vi "set_electrodes_init (SubVI).vi"(0 "Tot Electrode Arr":dbl[](array[numeric]), 5 "electrodes task 2":refnum<k21>, 9 "electrodes error":errorcluster, 11 "electrodes reference":refnum<vi>) -> (4 "electrode arr":dbl[][](array[numeric]), 6 "electrodes task":refnum<k21>, 15 "electrodes task error":errorcluster)   [LabVIEW 2018]
uses:
  <resource>/objmgr/daqmx.rc
  <vilib>/measure/NI_MABase.lvlib
panel:
  out "SampClk.Rate":dbl
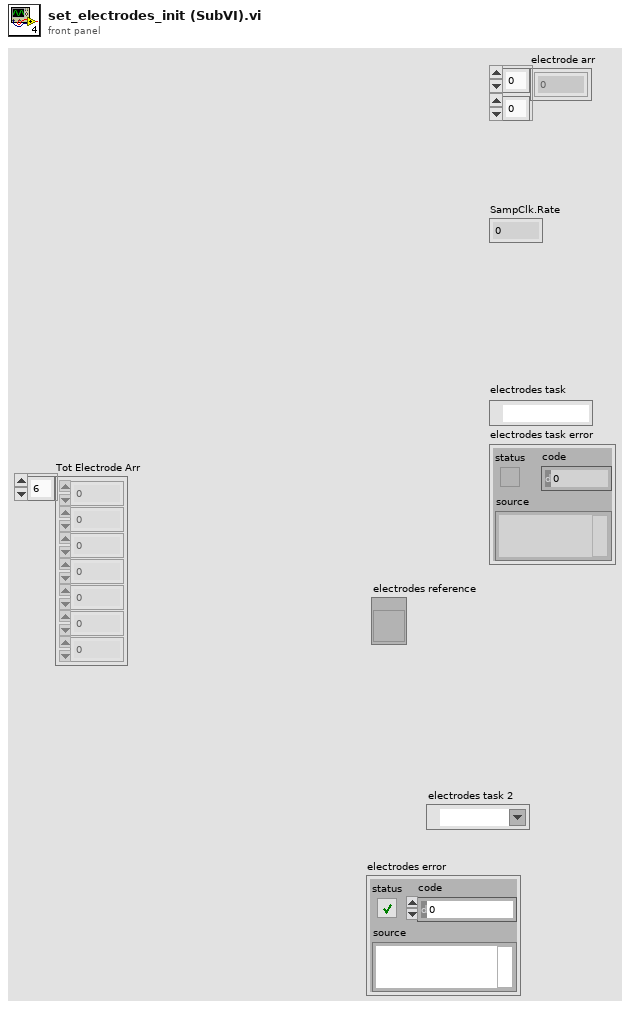
[diagram p1: front panel]
types:
  T1 = cluster{"DC volts (V):\n":dbl[], "Electrode to sweep:":i32, "start volt (V)":ext, "stop volt (V) ":ext, "# V Steps":i32, "start freq (Hz)":ext, "stop freq (Hz) ":ext, "# F steps":i32, "start DC (V)":ext, "stop DC (V)":ext, "# DC steps ":i32, "Digitize electrode\ndrives?":bool, "Sweep electrode?":bool, "Add 0.5*V DC \noffset for amp?":bool, "Use electrode \nconfig file?":bool, "Path":path, "Use arbitrary\nforce func?":bool, "Voltage vs pos file":path, "Use Arbitrary elec drive":bool, "Elec Drive File":path, "Filter Elecs?":bool, "Filter Cantilever?":bool, "Control DDS":bool}
  T2 = enum16{"Sine Wave", "Triangle Wave", "Square Wave", "Sawtooth Wave"}
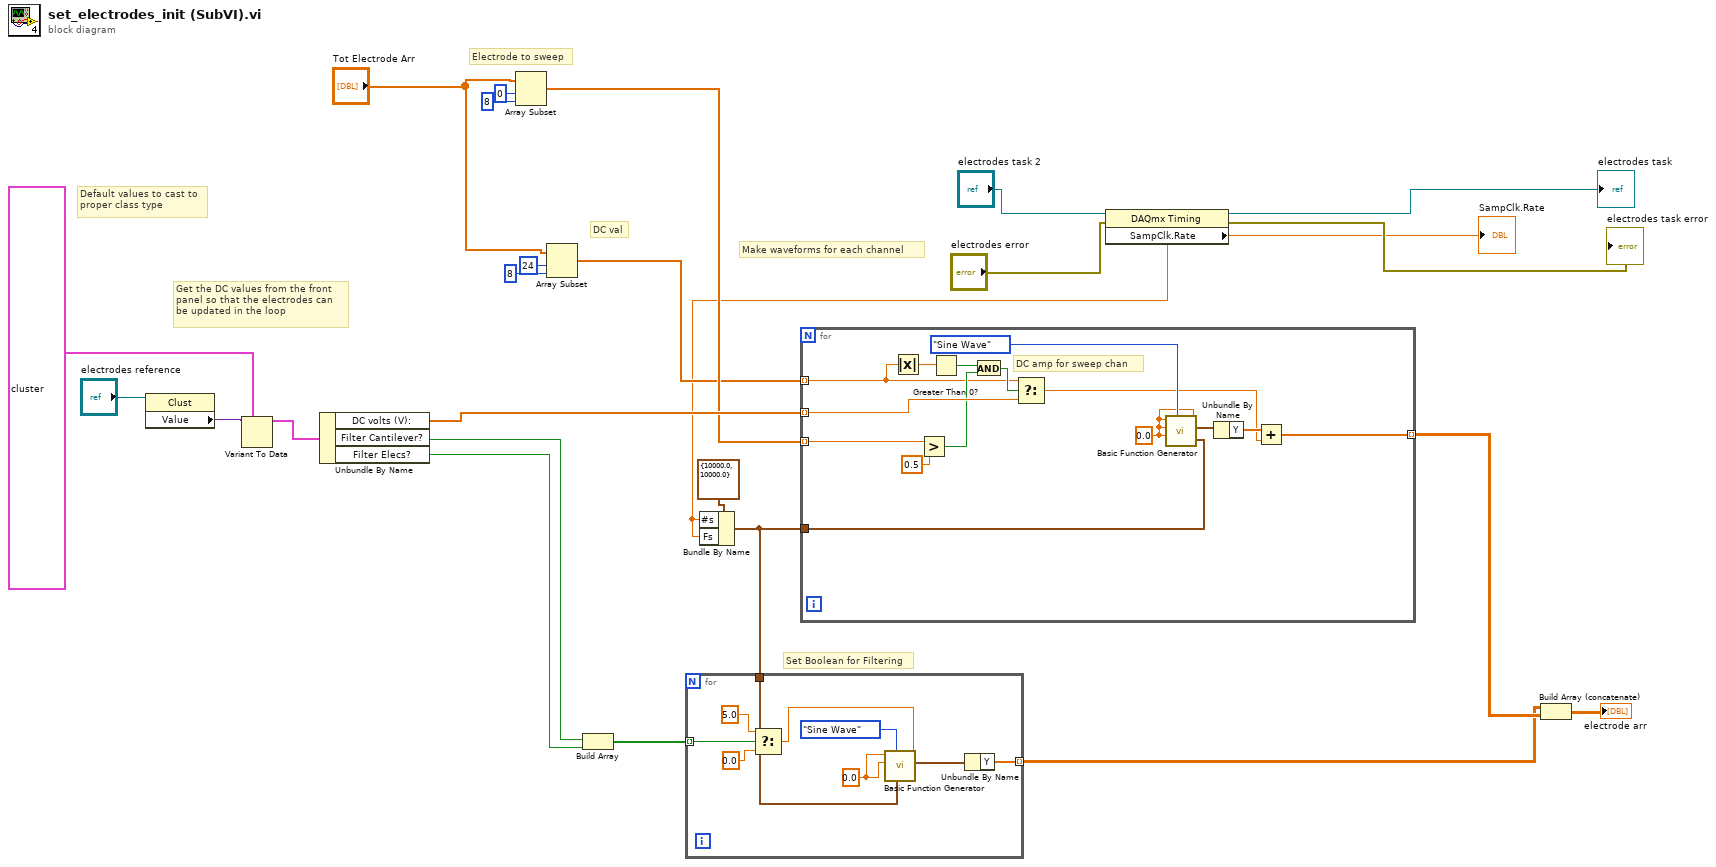
[diagram p0: block diagram]
diagram:
  # "Set Boolean for Filtering"
  # "Default values to cast to\nproper class type"
  # "Get the DC values from the front\npanel so that the electrodes can\nbe updated in the loop"
  # "Make waveforms for each channel"
  # "DC val"
  # "Electrode to sweep"
  n1 = property on="Property Node" class="Clust"(reference="electrodes reference") -> ("Value"=w19:variant)  [unwired: 1 in, 2 out]
  n2 = Variant To Data(type=T1 {"DC volts (V):\n"=[0.0, 0.0, 0.0, 0.0, 0.0, 0.0, 0.0, 0.0], "Electrode to sweep:"=3, "start volt (V)"=0.0, "stop volt (V) "=0.0, "# V Steps"=1, "start freq (Hz)"=41.0, "stop freq (Hz) "=41.0, "# F steps"=1, "start DC (V)"=0.0, "stop DC (V)"=0.0, "# DC steps "=1, "Digitize electrode\ndrives?"=TRUE, "Sweep electrode?"=FALSE, "Add 0.5*V DC \noffset for amp?"=FALSE, "Use electrode \nconfig file?"=FALSE, "Path"=path "", "Use arbitrary\nforce func?"=FALSE, "Voltage vs pos file"=path "", "Use Arbitrary elec drive"=FALSE, "Elec Drive File"=path "", "Filter Elecs?"=FALSE, "Filter Cantilever?"=FALSE, "Control DDS"=FALSE} ("Electrode settings:"), Variant=w19) -> (data=w18:T1)  [unwired: 1 in, 1 out]
  n3 = Unbundle By Name(w18) -> ("DC volts (V):"=w17:dbl[], "Filter Cantilever?"=w8:bool, "Filter Elecs?"=w7:bool)
  n4 = Array Subset(array="Tot Electrode Arr", index=0, length=8) -> (w14:dbl[])
  n5 = Array Subset(array="Tot Electrode Arr", index=24, length=8) -> (w13:dbl[])
  n6 = Build Array(w8, w7) -> (w6:bool[])
  n7 = property class="DAQmx Timing"(reference="electrodes task 2", error in="electrodes error") -> (reference out=→"electrodes task":refnum<k21>, error out=→"electrodes task error":errorcluster, "SampClk.Rate"=w2:dbl)
  "SampClk.Rate" <- w2
  n8 = Bundle By Name(cluster=cluster{"Fs":dbl, "#s":dbl} {"Fs"=10000.0, "#s"=10000.0} ("sampling info"), "#s"=w2, "Fs"=w2) -> (w9:cluster{"Fs":dbl, "#s":dbl})
  n9 = for {
    tunnel: w9 -> [w34]
    tunnel: w6 -> [w27] mode=indexing
    tunnel: [w26] -> w3 mode=indexing
    w31 = 0.0 ("f")
    n10 = Select(t=5.0 ("f"), s=w27, f=0.0) -> (s? t:f=w29:dbl)
    n11 = call <vilib>:"Basic Function Generator.vi"("offset"=w29, "sampling info"=w34, "signal type"=T2."Sine Wave", "amplitude"=w31, "frequency"=w31) -> ("signal out"=w28:waveform(dbl))  [unwired: 4 in, 2 out]
    n12 = Unbundle By Name(w28) -> ("Y"=w26:dbl[])
  }
  n13 = for {
    tunnel: w17 -> [w46] mode=indexing
    tunnel: w9 -> [w48]
    tunnel: [w39] -> w4 mode=indexing
    tunnel: w13 -> [w36] mode=indexing
    tunnel: w14 -> [w45] mode=indexing
    w35 = 0.0 ("y")
    # "DC amp for sweep chan"
    n14 = Absolute Value(x=w36) -> (abs(x)=w37:dbl)
    n15 = Greater?(x=w45, y=0.5) -> (0:w42:bool)
    n16 = Greater Than 0?(x=w37) -> (x > 0?=w38:bool)
    n17 = And(x=w38, y=w42) -> (x .and. y?=w43:bool)
    n18 = Select(t=w36, s=w43, f=w46) -> (s? t:f=w40:dbl)
    n19 = call <vilib>:"Basic Function Generator.vi"("offset"=w35, "sampling info"=w48, "signal type"=T2."Sine Wave", "phase"=w35, "amplitude"=w35, "frequency"=w35) -> ("signal out"=w47:waveform(dbl))  [unwired: 3 in, 2 out]
    n20 = Unbundle By Name(w47) -> ("Y"=w41:dbl[])
    n21 = Add(x=w41, y=w40) -> (x+y=w39:dbl[])
  }
  n22 = Build Array (concatenate)(w3, w4) -> (→"electrode arr":dbl[][])
